vi "Disconnect.vi"(8 "error in (no error)":errorcluster, 11 "Agilent DSO-X 3032A in":refnum<class "Agilent DSO-X 3032A.lvclass">) -> (0 "error out":errorcluster, 3 "Agilent DSO-X 3032A out":refnum<class "Agilent DSO-X 3032A.lvclass">)   [LabVIEW 2014, in "Agilent DSO-X 3032A.lvclass"]
uses:
  Agilent DSO-X 3032A.lvclass
  Agilent DSO-X 3032A.lvclass/Agilent DSO-X 3032A.ctl
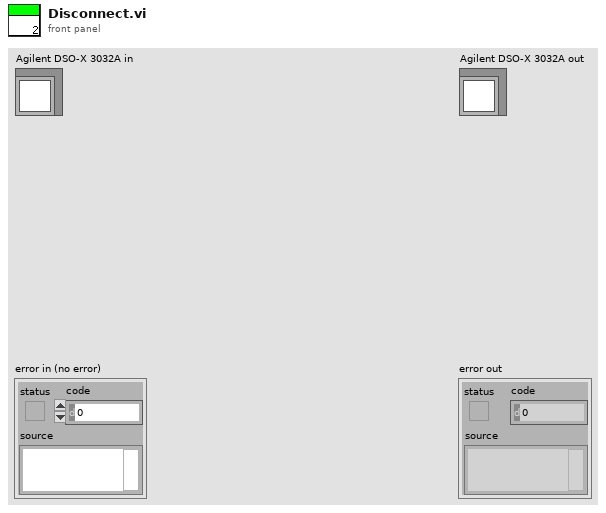
[diagram p1: front panel]
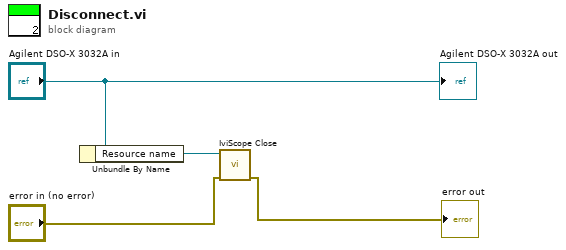
[diagram p0: block diagram]
diagram:
  n1 = Unbundle By Name("Agilent DSO-X 3032A in") -> ("Resource name"=w3:refnum<k15>)
  n2 = call <vilib>:"IviScope Close.vi"("error in (no error)"="error in (no error)", "instrument handle"=w3) -> ("error out"=→"error out":errorcluster)  [unwired: 9 out]
  "Agilent DSO-X 3032A out" <- "Agilent DSO-X 3032A in"
